vi "is_num.vi"(1 "char":u8) -> (0 "isNum":bool)   [LabVIEW 2011]
panel:
  out "string":string
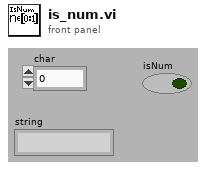
[diagram p1: front panel]
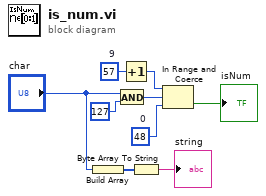
[diagram p0: block diagram]
diagram:
  w2 = u8 57  # 9
  w8 = u8 48  # 0
  n1 = Build Array("char") -> (w4:u8[])
  n2 = And(x="char", y=u8 127) -> (x .and. y?=w7:u8)
  n3 = Increment(x=w2) -> (x+1=w1:u8)
  n4 = Byte Array To String(unsigned byte array=w4) -> (string=→"string":string)
  n5 = In Range and Coerce(upper limit=w1, x=w7, lower limit=w8) -> (In Range?=→"isNum":bool)  [unwired: 1 out]
